vi "AdaptToInputs.vi"(3 "Term Types":T1, 4 "XRef":refnum<vi>, 5 "State In":T5) -> (0 "Reply":string[](array[string]), 2 "State Out":T5)   [LabVIEW 2012, in "OpenG Conditiional Auto-Indexing Tunnel.xnode"]
uses:
  OpenG Conditiional Auto-Indexing Tunnel.xnode
  State.ctl
  <vilib>/XNodeSupport/XNodeTermTypeIDPairs.ctl
  <vilib>/XNodeSupport/XNodeTermTypeIDPair.ctl
  <vilib>/XNodeSupport/XNodeType.ctl
  <vilib>/XNodeSupport/XNodeString.ctl
  <userlib>/_LAVAcr/Scripting Tools/XNode Support/TypeDefs/Array element Tests.ctl
  VI Scripting/Scripting Tools/XNode Support/Find term type by ID_type.vi
  VI Scripting/Scripting Tools/XNode Support/XNode Support.lvlib
  <vilib>/XNodeSupport/NI_XNodeSupport.lvlib
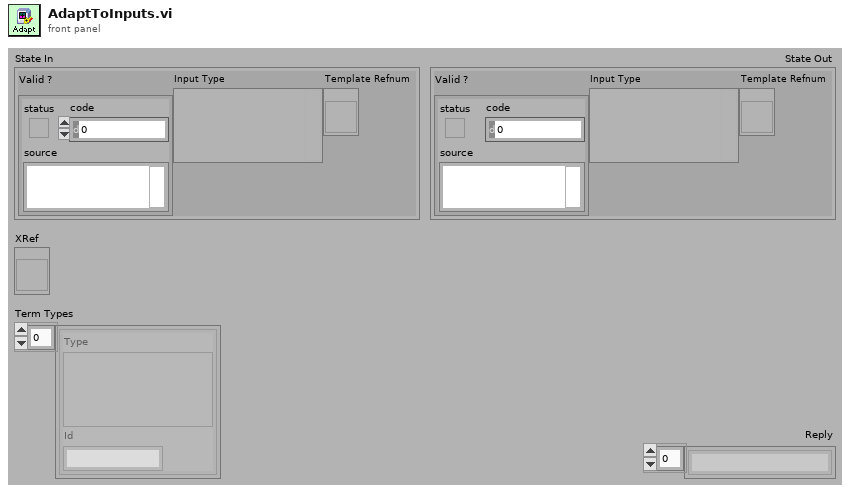
[diagram p1: front panel]
types:
  T1 = typedef "NI_XNodeSupport.lvlib/XNodeTermTypeIDPairs.ctl" = T2[]
  T2 = typedef "NI_XNodeSupport.lvlib/XNodeTermTypeIDPair.ctl" = cluster{"Type":T3, "Id":T4}
  T3 = typedef "NI_XNodeSupport.lvlib/XNodeType.ctl" = variant
  T4 = typedef "NI_XNodeSupport.lvlib/XNodeString.ctl" = string
  T5 = typedef "OpenG Conditiional Auto-Indexing Tunnel.xnode/State.ctl" = cluster{"Valid ?":errorcluster, "Input Type":variant, "Template Refnum":refnum<vi>}
  T6 = typedef "Scripting Tools.lvlib/XNode Support.lvlib/Array element Tests.ctl" = enum16{"Any Element", "Numeric", "Integer", "Float", "Complex", "Boolean", "String", "Sortable"}
  T7 = enum16{"No Check", "At Least n dimensions", "Exactly N Dimensions"}
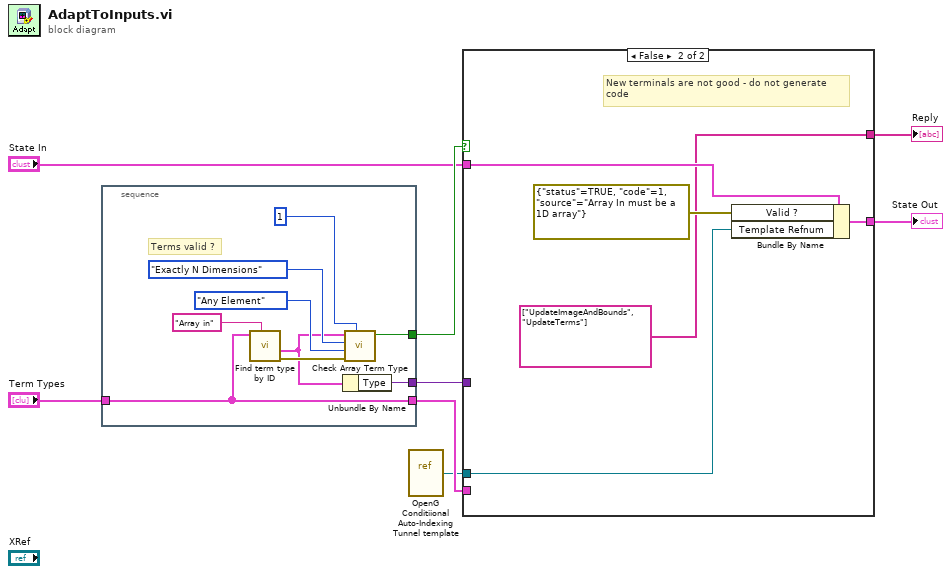
[diagram p0: block diagram]
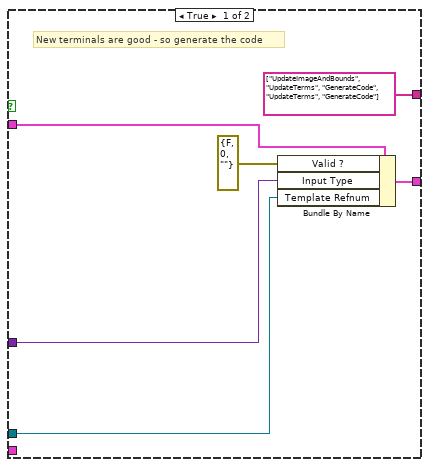
[diagram p2: hidden frame]
diagram:
  n1 = stacked-sequence {
    tunnel: "Term Types" -> [w17]
    tunnel: [w17] -> w6
    tunnel: [w9] -> w7
    tunnel: [w10] -> w2
    frame #0 {
      # "Terms valid ?"
      n2 = call-poly "Find term type by ID.vi"("Search ID"="Array in", "Term Types"=w17) -> ("error out"=w15:errorcluster, "Term Type"=w11:T2)  [unwired: 1 in, 7 out]
      n3 = Unbundle By Name(w11) -> ("Type"=w10:T3)
      n4 = call <userlib>:"Check Array Term Type.vi"("Dimensions Required"=1, "error in (no error)"=w15, "Element Check"=Array_element_Tests."Any Element", "Dimension Check"=T7."Exactly N Dimensions", "Term Type"=w11) -> ("Is Good ?"=w9:bool)  [unwired: 6 out]
    }
  }
  n5 = vi-ref "OpenG Conditiional Auto-Indexing Tunnel template.vi"() -> (w1:refnum<vi>)
  n6 = case shown="False" w7 {
    tunnel: w6 -> [_ _]
    tunnel: "State In" -> [w23 w28]
    tunnel: [w21 w26] -> w4
    tunnel: [string[] ["UpdateImageAndBounds", "UpdateTerms", "GenerateCode", "UpdateTerms", "GenerateCode"] ("Reply") string[] ["UpdateImageAndBounds", "UpdateTerms"] ("Reply")] -> w3
    tunnel: w2 -> [w19 _]
    tunnel: w1 -> [w18 w25]
    frame True {
      # "New terminals are good - so generate the code"
      n7 = Bundle By Name(cluster=w23, "Valid ?"=errorcluster {"status"=FALSE, "code"=0, "source"=""}, "Input Type"=w19, "Template Refnum"=w18) -> (w21:T5)
    }
    frame False {
      # "New terminals are not good - do not generate\ncode"
      n8 = Bundle By Name(cluster=w28, "Valid ?"=errorcluster {"status"=TRUE, "code"=1, "source"="Array In must be a 1D array"}, "Template Refnum"=w25) -> (w26:T5)
    }
  }
  "Reply" <- w3
  "State Out" <- w4
